vi "flattenAngularVelocityToXML_Array.vi"(8 "error in (no error)":errorcluster, 9 "angularVelocityUnitInXML":T1, 10 "angularVelocityAgain":variant, 11 "angularVelocity":dbl[unit][](array[numeric])) -> (0 "error out":errorcluster, 3 "xmlString":string)   [LabVIEW 2012, in "UnitsAndXML.lvlib"]
uses:
  <userlib>/Common/UnitsAndXML/UnitsAndXML.lvlib
  <userlib>/Common/UnitsAndXML/FlattenItemWithUnitToXML/FlattenAngularVelocityToXML/AngularVelocityUnit.ctl
  <vilib>/Utility/VariantDataType/VariantType.lvlib
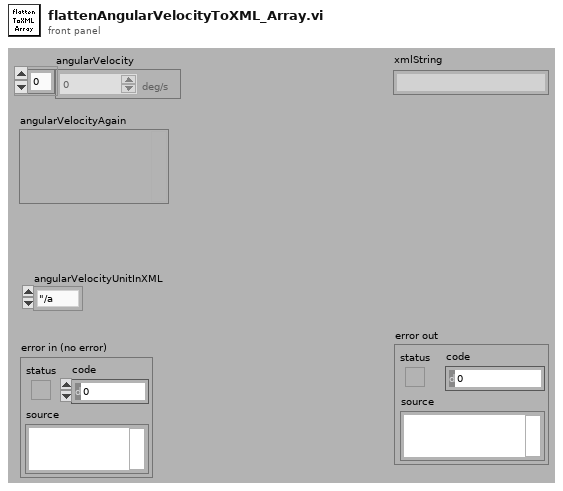
[diagram p1: front panel]
types:
  T1 = typedef "UnitsAndXML.lvlib/AngularVelocityUnit.ctl" = enum16{"\"/a", "deg/s", "\"/s"}
  T2 = typedef "VariantType.lvlib/Type.ctl" = enum8{"Invalid Type", "Void", "I8", "I16", "I32", "I64", "U8", "U16", "U32", "U64", "Single Float", "Double Float", "Extended Float", "Single Complex", "Double Complex", "Extended Complex", "Enum U8", "Enum U16", "Enum U32", "Enum U64", "Single Float With Unit", "Double Float With Unit", "Extended Float With Unit", "Single Complex with Unit", "Double Complex with Unit", "Extended Complex with Unit", "Boolean", "String", "Path", "Picture", "Tag", "Array", "Cluster", "Variant", "LV Variant", "Waveform", "Timestamp", "Digital Waveform", "Digital Data", "ExpressData", "Refnum", "External Data", "VI", "Poly VI", "LabVIEW Class Instance", "Fixed Point"}
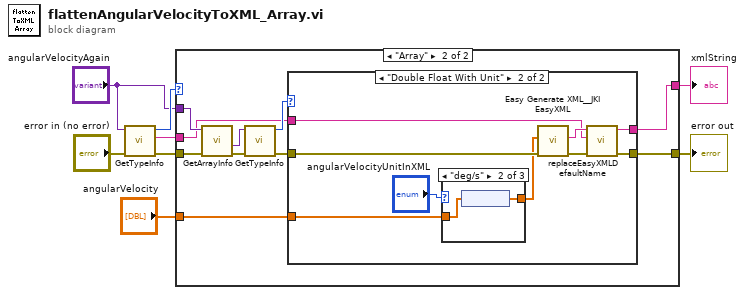
[diagram p0: block diagram]
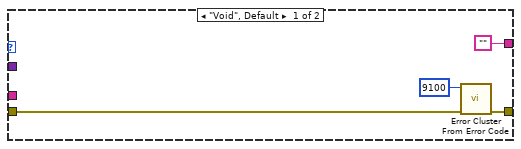
[diagram p2: hidden frame]
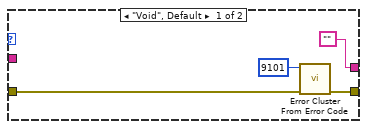
[diagram p3: hidden frame]
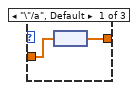
[diagram p4: hidden frame]
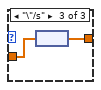
[diagram p5: hidden frame]
diagram:
  n1 = call <vilib>:"GetTypeInfo.vi"("error in (no error)"="error in (no error)", "Variant"="angularVelocityAgain") -> ("error out"=w2:errorcluster, "Name"=w1:string, "Type Enum"=w4:T2)  [unwired: 5 in, 2 out]
  n2 = case shown="\"Array\"" w4 {
    tunnel: "angularVelocity" -> [_ w18]
    tunnel: ["" w16] -> w7
    tunnel: [w9 w17] -> w6
    tunnel: "angularVelocityAgain" -> [_ w22]
    tunnel: w2 -> [w10 w15]
    tunnel: w1 -> [_ w13]
    frame "Void", Default {
      n3 = call <vilib>:"Error Cluster From Error Code.vi"("error in (no error)"=w10, "error code (0)"=9100) -> ("error out"=w9:errorcluster)  [unwired: 7 in]
    }
    frame "Array" {
      n4 = call <vilib>:"GetArrayInfo.vi"("error in (no error)"=w15, "Variant"=w22) -> ("error out"=w21:errorcluster, "ArrayElement"=w20:variant)  [unwired: 6 in, 2 out]
      n5 = call <vilib>:"GetTypeInfo.vi"("error in (no error)"=w21, "Variant"=w20) -> ("error out"=w14:errorcluster, "Type Enum"=w19:T2)  [unwired: 5 in, 3 out]
      n6 = case shown="\"Double Float With Unit\"" w19 {
        tunnel: w18 -> [_ w28]
        tunnel: ["" w34] -> w16
        tunnel: [w23 w33] -> w17
        tunnel: w14 -> [w24 w32]
        tunnel: w13 -> [_ w30]
        frame "Void", Default {
          n7 = call <vilib>:"Error Cluster From Error Code.vi"("error in (no error)"=w24, "error code (0)"=9101) -> ("error out"=w23:errorcluster)  [unwired: 7 in]
        }
        frame "Double Float With Unit" {
          n8 = case shown="\"deg/s\"" "angularVelocityUnitInXML" {
            tunnel: w28 -> [w37 w39 w41]
            tunnel: [w36 w38 w40] -> w27
            frame "\"/a", Default {
              n9 = node(w37) -> (w36:dbl[])
            }
            frame "deg/s" {
              n10 = node(w39) -> (w38:dbl[])
            }
            frame "\"/s" {
              n11 = node(w41) -> (w40:dbl[])
            }
          }
          n12 = call <vilib>:"Easy Generate XML__JKI EasyXML.vi"("error in (no error)"=w32, "LabVIEW Data"=w27) -> ("error out"=w31:errorcluster, "XML String"=w35:string)  [unwired: 8 in]
          n13 = call <userlib>:"replaceEasyXMLDefaultName.vi"("error in"=w31, "desiredName"=w30, "easyXMLStringWithDefaultNames"=w35) -> ("error out"=w33:errorcluster, "xmlString"=w34:string)  [unwired: 7 in]
        }
      }
    }
  }
  "xmlString" <- w7
  "error out" <- w6
